vi "Insert Panel.vi"(8 "error in (no error)":errorcluster, 11 "Abstruct View in":refnum<class "Abstruct View.lvclass">) -> (0 "error out":errorcluster, 3 "Abstruct View out":refnum<class "Abstruct View.lvclass">)   [LabVIEW 2020, in "Abstruct View.lvlib" / "Abstruct View.lvclass"]
uses:
  Abstruct View.lvclass
  Abstruct View.lvclass/Abstruct View.ctl
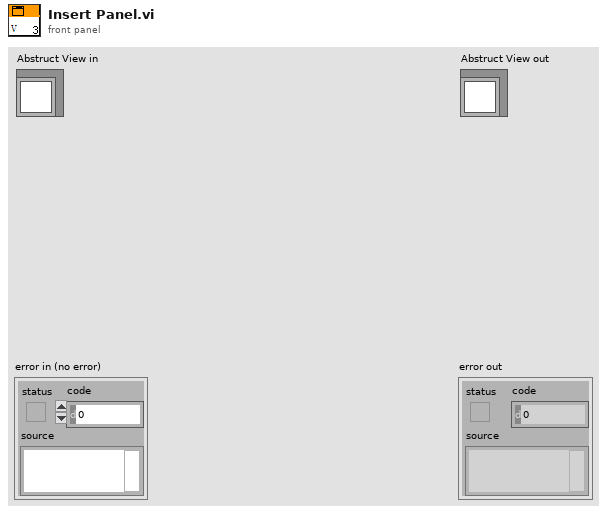
[diagram p1: front panel]
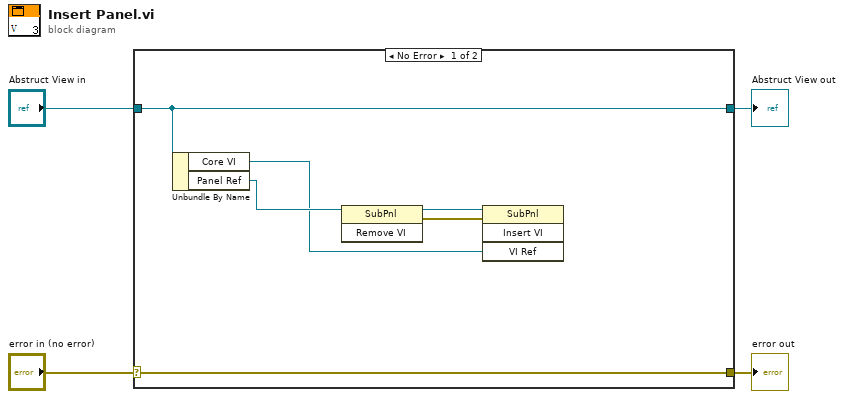
[diagram p0: block diagram]
diagram:
  n1 = case shown="No Error" "error in (no error)" {
    selector: "error in (no error)" -> [w10 w12]
    tunnel: [w10 w12] -> w3
    tunnel: [w9 w11] -> w1
    tunnel: "Abstruct View in" -> [w9 w11]
    frame No Error {
      n2 = Unbundle By Name(w9) -> ("Core VI"=w5:refnum<vi>, "Panel Ref"=w6:refnum<vi>)
      n3 = invoke class="SubPnl" method="Remove VI"(reference=w6) -> (reference out=w8:refnum<vi>, error out=w7:errorcluster)  [unwired: 2 in, 1 out]
      n4 = invoke class="SubPnl" method="Insert VI"(reference=w8, error in=w7, "VI Ref"=w5) -> ()  [unwired: 1 in, 4 out]
    }
    frame Error {
    }
  }
  "error out" <- w3
  "Abstruct View out" <- w1
